vi "PromptSetup.vi"(11 "Email Notification Cluster IN":T1) -> (3 "Email Notification Cluster OUT":T1)   [LabVIEW 2012]
uses:
  Archive and FTP Software/Controls/Ping address and email notify.ctl
panel:
  in  "Email Notification SET":T1
  in  "OK Button":bool
  in  "Cancel Button":bool
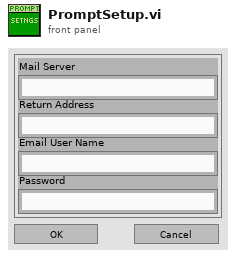
[diagram p1: front panel]
types:
  T1 = typedef "Ping address and email notify.ctl" = cluster{"Mail Server":string, "Return Address":string, "Email User Name":string, "Password":string}
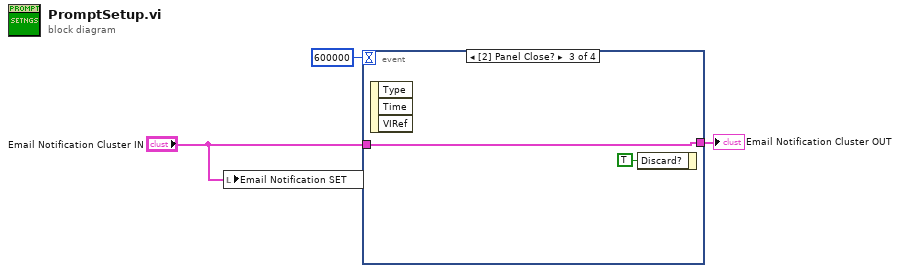
[diagram p0: block diagram]
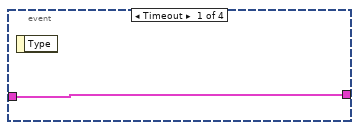
[diagram p2: hidden frame]
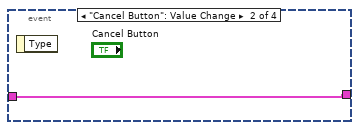
[diagram p3: hidden frame]
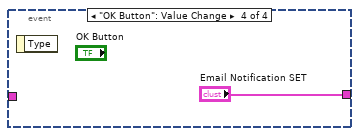
[diagram p4: hidden frame]
diagram:
  n1 = local write "Email Notification SET"("Email Notification Cluster IN") -> ()
  n2 = event shown="[2] Panel Close?" {
    selector: _ -> [_ _ _ _]
    dyn-events: _ -> [_ _ _ _]
    timeout: 600000 -> [_ _ _ _]
    tunnel: "Email Notification Cluster IN" -> [w4 w5 w6 _]
    tunnel: [w4 w5 w6 "Email Notification SET"] -> w2
    event Timeout {
      n3 = event-data() -> ()  [unwired: 1 in, 1 out]
    }
    event "Cancel Button": Value Change {
      n4 = event-data() -> ()  [unwired: 1 in, 1 out]
    }
    event Panel Close? {
      n5 = event-data() -> ()  [unwired: 1 in, 3 out]
      n6 = event-data("Discard?"=TRUE) -> ()  [unwired: 1 in, 1 out]
    }
    event "OK Button": Value Change {
      n7 = event-data() -> ()  [unwired: 1 in, 1 out]
    }
  }
  "Email Notification Cluster OUT" <- w2
